vi "Send_CAN_ATII.vi"(0 "MsgTX":T1 {"MSGTYPE" items=["STATUS"=128, "EXTENDED"=2, "RTR"=1, "DATA MSG"=0]}, 1 "Config":refnum<vi>) -> ()   [LabVIEW 2010]
uses:
  PCAN_Driver/ControlCAN.llb/VCI_CAN_OBJ.ctl
  PCAN_Driver/ControlCAN.lvlib
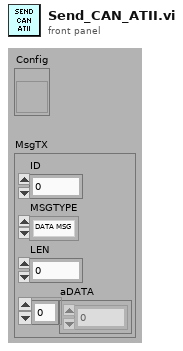
[diagram p1: front panel]
types:
  T1 = cluster{"ID":u32, "MSGTYPE":u8, "LEN":u8, "aDATA":u8[]}
  T2 = typedef "ControlCAN.lvlib/VCI_CAN_OBJ.ctl" = cluster{"ID":u32, "TimeStamp":u32, "TimeFlag":u8, "SendType":u8, "RemoteFlag":u8, "ExternFlag":u8, "DataLen":u8, "Data":u8[], "Reserved":u8[]}
  T3 = typedef "ControlCAN.lvlib/DevType.ctl" = u32
  T4 = typedef "ControlCAN.lvlib/CAN Channel.ctl" = u32
  T5 = typedef "ControlCAN.lvlib/VCI_INIT_CONFIG.ctl" = cluster{"AccCode":u32, "AccMask":u32, "InitFlag":T6, "Fliter":T7, "Timing0":u8, "Timing1":u8, "Mode":T8}
  T6 = typedef "ControlCAN.lvlib/InitFlag.ctl" = u32
  T7 = typedef "ControlCAN.lvlib/Fliter.ctl" = u8
  T8 = typedef "ControlCAN.lvlib/Mode.ctl" = u8
  T9 = cluster{"DevType":T3, "DevIndex":u32, "CanIndex":T4, "VCI_INIT_CONFIG":T5}
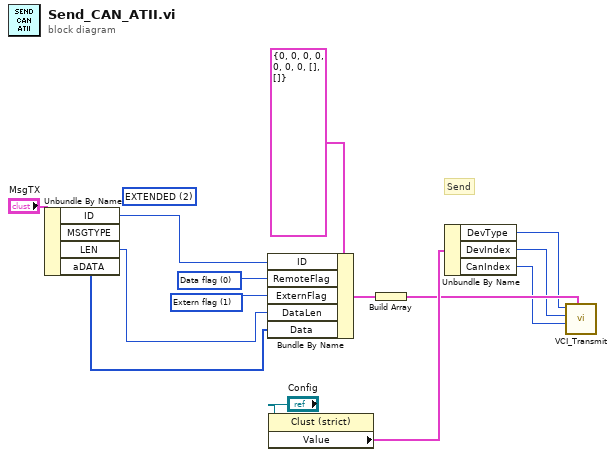
[diagram p0: block diagram]
diagram:
  (unwired) u8 2 items=["STATUS"=128, "EXTENDED"=2, "RTR"=1, "DATA MSG"=0] ("MSGTYPE")
  w3 = u8 1 items=["Standart flag", "Extern flag"] ("Format")
  w2 = u8 0 items=["Data flag", "Remote flag"] ("Type")
  # "Send"
  n1 = Unbundle By Name("MsgTX") -> ("ID"=w12:u32, "LEN"=w13:u8, "aDATA"=w14:u8[])  [unwired: 1 out]
  n2 = Bundle By Name(cluster=T2 {"ID"=0, "TimeStamp"=0, "TimeFlag"=0, "SendType"=0, "RemoteFlag"=0, "ExternFlag"=0, "DataLen"=0, "Data"=[], "Reserved"=[]} ("Send"), "ID"=w12, "RemoteFlag"=w2, "ExternFlag"=w3, "DataLen"=w13, "Data"=w14) -> (w8:T2)
  n3 = property class="Clust (strict)"(reference="Config") -> ("Value"=w10:T9)  [unwired: 1 in, 2 out]
  n4 = Build Array(w8) -> (w7:T2[])
  n5 = Unbundle By Name(w10) -> ("DevType"=w4:T3, "DevIndex"=w5:u32, "CanIndex"=w6:T4)
  n6 = call "VCI_Transmit.vi"("Buffer"=w7, "CANIndex"=w6, "DevIndex"=w5, "DevType"=w4) -> ()  [unwired: 1 in, 7 out]
